vi "nanocal -- nuclear schottky fit V7.vi"() -> ()   [LabVIEW 2021] (continued)
0.000000000000   ,  \"Imoff\" -> 0.000000000000   ,  \"στ1\" -> 0.000000000000   ,  \"στS\" -> 0.000000000000   ,  \"στN\" -> 0.000000000000    |>   , \n\"IDS0531_220605_RAW_cal__ref_\" ->   <|    \"ζ\" -> 0.047292360430   ,  \"τ1\" -> 0.215650832524   ,  \"τS\" -> 0.021748628873   ,  \"τN\" -> 0.002014257649   ,  \"τC\" -> 0.001656178311   ,  \"κ0\" -> 0.000000003034   ,  \"mm1\" -> 0.000069918264   ,  \"mm2\" -> 0.024098100915   ,  \"mm3\" -> 0.218025681173   ,  \"T\" -> 0.520000000000   ,  \"B\" -> 4.000000000000   ,  \"θ\" -> 45.000000000000   ,  \"Reoff\" -> -2955102.040816321970   ,  \"Imoff\" -> 0.000000000000   ,  \"στ1\" -> 0.046963197390   ,  \"στS\" -> 0.000145543572   ,  \"στN\" -> 0.000181922698    |>   , \n\"IDS0531_220605_RAW_cal__sam_\" ->   <|    \"ζ\" -> 0.000000000000   ,  \"τ1\" -> 0.000000000000   ,  \"τS\" -> 0.000000000000   ,  \"τN\" -> 0.000000000000   ,  \"τC\" -> 0.000000000000   ,  \"κ0\" -> 0.000000000000   ,  \"mm1\" -> 0.000000000000   ,  \"mm2\" -> 0.000000000000   ,  \"mm3\" -> 0.000000000000   ,  \"T\" -> 0.520000000000   ,  \"B\" -> 4.000000000000   ,  \"θ\" -> 45.000000000000   ,  \"Reoff\" -> 0.000000000000   ,  \"Imoff\" -> 0.000000000000   ,  \"στ1\" -> 0.000000000000   ,  \"στS\" -> 0.000000000000   ,  \"στN\" -> 0.000000000000    |>   , \n\"IDS0532_220605_RAW_cal__ref_\" ->   <|    \"ζ\" -> 0.039581980273   ,  \"τ1\" -> 0.217269361754   ,  \"τS\" -> 0.023071327438   ,  \"τN\" -> 0.001182618434   ,  \"τC\" -> 0.001652851775   ,  \"κ0\" -> 0.000000003717   ,  \"mm1\" -> 0.000059010683   ,  \"mm2\" -> 0.025415535832   ,  \"mm3\" -> 0.218661632092   ,  \"T\" -> 0.620000000000   ,  \"B\" -> 4.000000000000   ,  \"θ\" -> 45.000000000000   ,  \"Reoff\" -> -2746938.775510199370   ,  \"Imoff\" -> 0.000000000000   ,  \"στ1\" -> 0.015098698436   ,  \"στS\" -> 0.000189797573   ,  \"στN\" -> 0.000008998512    |>   , \n\"IDS0532_220605_RAW_cal__sam_\" ->   <|    \"ζ\" -> 0.000000000000   ,  \"τ1\" -> 0.000000000000   ,  \"τS\" -> 0.000000000000   ,  \"τN\" -> 0.000000000000   ,  \"τC\" -> 0.000000000000   ,  \"κ0\" -> 0.000000000000   ,  \"mm1\" -> 0.000000000000   ,  \"mm2\" -> 0.000000000000   ,  \"mm3\" -> 0.000000000000   ,  \"T\" -> 0.620000000000   ,  \"B\" -> 4.000000000000   ,  \"θ\" -> 45.000000000000   ,  \"Reoff\" -> 0.000000000000   ,  \"Imoff\" -> 0.000000000000   ,  \"στ1\" -> 0.000000000000   ,  \"στS\" -> 0.000000000000   ,  \"στN\" -> 0.000000000000    |>   , \n\"IDS0533_220605_RAW_cal__ref_\" ->   <|    \"ζ\" -> 0.026006399704   ,  \"τ1\" -> 0.219491604326   ,  \"τS\" -> 0.026508960211   ,  \"τN\" -> 0.000691251356   ,  \"τC\" -> 0.002192117759   ,  \"κ0\" -> 0.000000005099   ,  \"mm1\" -> 0.000051510023   ,  \"mm2\" -> 0.029230026409   ,  \"mm3\" -> 0.220309776794   ,  \"T\" -> 0.820000000000   ,  \"B\" -> 4.000000000000   ,  \"θ\" -> 45.000000000000   ,  \"Reoff\" -> -873469.387755103408   ,  \"Imoff\" -> 0.000000000000   ,  \"στ1\" -> 0.040897544111   ,  \"στS\" -> 0.000189265066   ,  \"στN\" -> 0.000022111002    |>   , \n\"IDS0533_220605_RAW_cal__sam_\" ->   <|    \"ζ\" -> 0.000000000000   ,  \"τ1\" -> 0.000000000000   ,  \"τS\" -> 0.000000000000   ,  \"τN\" -> 0.000000000000   ,  \"τC\" -> 0.000000000000   ,  \"κ0\" -> 0.000000000000   ,  \"mm1\" -> 0.000000000000   ,  \"mm2\" -> 0.000000000000   ,  \"mm3\" -> 0.000000000000   ,  \"T\" -> 0.820000000000   ,  \"B\" -> 4.000000000000   ,  \"θ\" -> 45.000000000000   ,  \"Reoff\" -> 0.000000000000   ,  \"Imoff\" -> 0.000000000000   ,  \"στ1\" -> 0.000000000000   ,  \"στS\" -> 0.000000000000   ,  \"στN\" -> 0.000000000000    |>   , \n\"IDS0534_220605_RAW_cal__ref_\" ->   <|    \"ζ\" -> 0.022451049934   ,  \"τ1\" -> 0.221358754558   ,  \"τS\" -> 0.033966694492   ,  \"τN\" -> 0.000363309481   ,  \"τC\" -> 0.002245679298   ,  \"κ0\" -> 0.000000007138   ,  \"mm1\" -> 0.000046374039   ,  \"mm2\" -> 0.036854393963   ,  \"mm3\" -> 0.221804414461   ,  \"T\" -> 1.120000000000   ,  \"B\" -> 4.000000000000   ,  \"θ\" -> 45.000000000000   ,  \"Reoff\" -> -885714.285714285447   ,  \"Imoff\" -> 0.000000000000   ,  \"στ1\" -> 0.023144908767   ,  \"στS\" -> 0.000217300505   ,  \"στN\" -> 0.000007634517    |>   , \n\"IDS0534_220605_RAW_cal__sam_\" ->   <|    \"ζ\" -> 0.000000000000   ,  \"τ1\" -> 0.000000000000   ,  \"τS\" -> 0.000000000000   ,  \"τN\" -> 0.000000000000   ,  \"τC\" -> 0.000000000000   ,  \"κ0\" -> 0.000000000000   ,  \"mm1\" -> 0.000000000000   ,  \"mm2\" -> 0.000000000000   ,  \"mm3\" -> 0.000000000000   ,  \"T\" -> 1.120000000000   ,  \"B\" -> 4.000000000000   ,  \"θ\" -> 45.000000000000   ,  \"Reoff\" -> 0.000000000000   ,  \"Imoff\" -> 0.000000000000   ,  \"στ1\" -> 0.000000000000   ,  \"στS\" -> 0.000000000000   ,  \"στN\" -> 0.000000000000    |>   , \n\"IDS0535_220605_RAW_cal__ref_\" ->   <|    \"ζ\" -> 0.019576865757   ,  \"τ1\" -> 0.218088277374   ,  \"τS\" -> 0.022473990539   ,  \"τN\" -> 0.000172254737   ,  \"τC\" -> 0.002442141955   ,  \"κ0\" -> 0.000000011417   ,  \"mm1\" -> 0.000042446249   ,  \"mm2\" -> 0.025290622371   ,  \"mm3\" -> 0.218286938488   ,  \"T\" -> 1.700000000000   ,  \"B\" -> 4.000000000000   ,  \"θ\" -> 45.000000000000   ,  \"Reoff\" -> -322448.979591836221   ,  \"Imoff\" -> 0.000000000000   ,  \"στ1\" -> 0.063627358635   ,  \"στS\" -> 0.000720787697   ,  \"στN\" -> 0.000014224220    |>   , \n\"IDS0535_220605_RAW_cal__sam_\" ->   <|    \"ζ\" -> 0.000000000000   ,  \"τ1\" -> 0.000000000000   ,  \"τS\" -> 0.000000000000   ,  \"τN\" -> 0.000000000000   ,  \"τC\" -> 0.000000000000   ,  \"κ0\" -> 0.000000000000   ,  \"mm1\" -> 0.000000000000   ,  \"mm2\" -> 0.000000000000   ,  \"mm3\" -> 0.000000000000   ,  \"T\" -> 1.700000000000   ,  \"B\" -> 4.000000000000   ,  \"θ\" -> 45.000000000000   ,  \"Reoff\" -> 0.000000000000   ,  \"Imoff\" -> 0.000000000000   ,  \"στ1\" -> 0.000000000000   ,  \"στS\" -> 0.000000000000   ,  \"στN\" -> 0.000000000000    |>   , \n\"IDS0536_220605_RAW_cal__ref_\" ->   <|    \"ζ\" -> 0.017203827920   ,  \"τ1\" -> 0.213925239716   ,  \"τS\" -> 0.013557235716   ,  \"τN\" -> 0.000118116880   ,  \"τC\" -> 0.002620828700   ,  \"κ0\" -> 0.000000012687   ,  \"mm1\" -> 0.000037331962   ,  \"mm2\" -> 0.016364021106   ,  \"mm3\" -> 0.214055336357   ,  \"T\" -> 1.900000000000   ,  \"B\" -> 4.000000000000   ,  \"θ\" -> 45.000000000000   ,  \"Reoff\" -> -322448.979591836221   ,  \"Imoff\" -> 0.000000000000   ,  \"στ1\" -> 0.007920167579   ,  \"στS\" -> 0.000110474044   ,  \"στN\" -> 0.000002075732    |>   , \n\"IDS0536_220605_RAW_cal__sam_\" ->   <|    \"ζ\" -> 0.000000000000   ,  \"τ1\" -> 0.000000000000   ,  \"τS\" -> 0.000000000000   ,  \"τN\" -> 0.000000000000   ,  \"τC\" -> 0.000000000000   ,  \"κ0\" -> 0.000000000000   ,  \"mm1\" -> 0.000000000000   ,  \"mm2\" -> 0.000000000000   ,  \"mm3\" -> 0.000000000000   ,  \"T\" -> 1.900000000000   ,  \"B\" -> 4.000000000000   ,  \"θ\" -> 45.000000000000   ,  \"Reoff\" -> 0.000000000000   ,  \"Imoff\" -> 0.000000000000   ,  \"στ1\" -> 0.000000000000   ,  \"στS\" -> 0.000000000000   ,  \"στN\" -> 0.000000000000    |>   , \n\"IDS0537_220605_RAW_cal__ref_\" ->   <|    \"ζ\" -> 0.016837588937   ,  \"τ1\" -> 0.214083726987   ,  \"τS\" -> 0.009462256875   ,  \"τN\" -> 0.000044961797   ,  \"τC\" -> 0.002520072033   ,  \"κ0\" -> 0.000000022492   ,  \"mm1\" -> 0.000033158698   ,  \"mm2\" -> 0.012105753537   ,  \"mm3\" -> 0.214132184097   ,  \"T\" -> 3.100000000000   ,  \"B\" -> 4.000000000000   ,  \"θ\" -> 45.000000000000   ,  \"Reoff\" -> -200000.000000000000   ,  \"Imoff\" -> 0.000000000000   ,  \"στ1\" -> 0.041355363203   ,  \"στS\" -> 0.000204828997   ,  \"στN\" -> 0.000003281967    |>   , \n\"IDS0537_220605_RAW_cal__sam_\" ->   <|    \"ζ\" -> 0.000000000000   ,  \"τ1\" -> 0.000000000000   ,  \"τS\" -> 0.000000000000   ,  \"τN\" -> 0.000000000000   ,  \"τC\" -> 0.000000000000   ,  \"κ0\" -> 0.000000000000   ,  \"mm1\" -> 0.000000000000   ,  \"mm2\" -> 0.000000000000   ,  \"mm3\" -> 0.000000000000   ,  \"T\" -> 3.100000000000   ,  \"B\" -> 4.000000000000   ,  \"θ\" -> 45.000000000000   ,  \"Reoff\" -> 0.000000000000   ,  \"Imoff\" -> 0.000000000000   ,  \"στ1\" -> 0.000000000000   ,  \"στS\" -> 0.000000000000   ,  \"στN\" -> 0.000000000000    |>   , \n\"IDS0538_220605_RAW_cal__ref_\" ->   <|    \"ζ\" -> 0.019986975905   ,  \"τ1\" -> 0.213955272188   ,  \"τS\" -> 0.005937059985   ,  \"τN\" -> 0.000017131866   ,  \"τC\" -> 0.001979607590   ,  \"κ0\" -> 0.000000055230   ,  \"mm1\" -> 0.000029341516   ,  \"mm2\" -> 0.008005311507   ,  \"mm3\" -> 0.213973424895   ,  \"T\" -> 5.700000000000   ,  \"B\" -> 4.000000000000   ,  \"θ\" -> 45.000000000000   ,  \"Reoff\" -> -77551.020408162847   ,  \"Imoff\" -> 0.000000000000   ,  \"στ1\" -> 0.013237190857   ,  \"στS\" -> 0.000032983186   ,  \"στN\" -> 0.000000229969    |>   , \n\"IDS0538_220605_RAW_cal__sam_\" ->   <|    \"ζ\" -> 0.000000000000   ,  \"τ1\" -> 0.000000000000   ,  \"τS\" -> 0.000000000000   ,  \"τN\" -> 0.000000000000   ,  \"τC\" -> 0.000000000000   ,  \"κ0\" -> 0.000000000000   ,  \"mm1\" -> 0.000000000000   ,  \"mm2\" -> 0.000000000000   ,  \"mm3\" -> 0.000000000000   ,  \"T\" -> 5.700000000000   ,  \"B\" -> 4.000000000000   ,  \"θ\" -> 45.000000000000   ,  \"Reoff\" -> 0.000000000000   ,  \"Imoff\" -> 0.000000000000   ,  \"στ1\" -> 0.000000000000   ,  \"στS\" -> 0.000000000000   ,  \"στN\" -> 0.000000000000    |>   , \n\"IDS0540_220605_RAW_cal__ref_\" ->   <|    \"ζ\" -> 0.251392330354   ,  \"τ1\" -> 0.346377607558   ,  \"τS\" -> 0.016513842206   ,  \"τN\" -> 0.014262469720   ,  \"τC\" -> 0.000857308117   ,  \"κ0\" -> 0.000000000886   ,  \"mm1\" -> 0.000166652692   ,  \"mm2\" -> 0.020248144591   ,  \"mm3\" -> 0.365333359092   ,  \"T\" -> 0.200000000000   ,  \"B\" -> 2.000000000000   ,  \"θ\" -> 45.000000000000   ,  \"Reoff\" -> -46204081.632653057600   ,  \"Imoff\" -> 0.000000000000   ,  \"στ1\" -> 0.424749382693   ,  \"στS\" -> 0.000332071104   ,  \"στN\" -> 0.013507044944    |>   , \n\"IDS0540_220605_RAW_cal__sam_\" ->   <|    \"ζ\" -> 0.000000000000   ,  \"τ1\" -> 0.000000000000   ,  \"τS\" -> 0.000000000000   ,  \"τN\" -> 0.000000000000   ,  \"τC\" -> 0.000000000000   ,  \"κ0\" -> 0.000000000000   ,  \"mm1\" -> 0.000000000000   ,  \"mm2\" -> 0.000000000000   ,  \"mm3\" -> 0.000000000000   ,  \"T\" -> 0.200000000000   ,  \"B\" -> 2.000000000000   ,  \"θ\" -> 45.000000000000   ,  \"Reoff\" -> 0.000000000000   ,  \"Imoff\" -> 0.000000000000   ,  \"στ1\" -> 0.000000000000   ,  \"στS\" -> 0.000000000000   ,  \"στN\" -> 0.000000000000    |>   , \n\"IDS0541_220605_RAW_cal__ref_\" ->   <|    \"ζ\" -> 0.165113897347   ,  \"τ1\" -> 0.387980452993   ,  \"τS\" -> 0.014374929410   ,  \"τN\" -> 0.009383556190   ,  \"τC\" -> 0.000942269686   ,  \"κ0\" -> 0.000000001199   ,  \"mm1\" -> 0.000127336399   ,  \"mm2\" -> 0.017060680127   ,  \"mm3\" -> 0.399416047906   ,  \"T\" -> 0.250000000000   ,  \"B\" -> 2.000000000000   ,  \"θ\" -> 45.000000000000   ,  \"Reoff\" -> -23306122.448979616200   ,  \"Imoff\" -> 0.000000000000   ,  \"στ1\" -> 0.067668625614   ,  \"στS\" -> 0.000112915267   ,  \"στN\" -> 0.002227405906    |>   , \n\"IDS0541_220605_RAW_cal__sam_\" ->   <|    \"ζ\" -> 0.000000000000   ,  \"τ1\" -> 0.000000000000   ,  \"τS\" -> 0.000000000000   ,  \"τN\" -> 0.000000000000   ,  \"τC\" -> 0.000000000000   ,  \"κ0\" -> 0.000000000000   ,  \"mm1\" -> 0.000000000000   ,  \"mm2\" -> 0.000000000000   ,  \"mm3\" -> 0.000000000000   ,  \"T\" -> 0.250000000000   ,  \"B\" -> 2.000000000000   ,  \"θ\" -> 45.000000000000   ,  \"Reoff\" -> 0.000000000000   ,  \"Imoff\" -> 0.000000000000   ,  \"στ1\" -> 0.000000000000   ,  \"στS\" -> 0.000000000000   ,  \"στN\" -> 0.000000000000    |>   , \n\"IDS0542_220606_RAW_cal__ref_\" ->   <|    \"ζ\" -> 0.345710784026   ,  \"τ1\" -> 0.327857477320   ,  \"τS\" -> 0.019203362427   ,  \"τN\" -> 0.016889536551   ,  \"τC\" -> 0.000830598267   ,  \"κ0\" -> 0.000000000695   ,  \"mm1\" -> 0.000208359489   ,  \"mm2\" -> 0.024619495516   ,  \"mm3\" -> 0.352430823963   ,  \"T\" -> 0.170000000000   ,  \"B\" -> 2.000000000000   ,  \"θ\" -> 45.000000000000   ,  \"Reoff\" -> -73265306.122448980800   ,  \"Imoff\" -> 0.000000000000   ,  \"στ1\" -> 0.369953882310   ,  \"στS\" -> 0.000610690630   ,  \"στN\" -> 0.016945730597    |>   , \n\"IDS0542_220606_RAW_cal__sam_\" ->   <|    \"ζ\" -> 0.000000000000   ,  \"τ1\" -> 0.000000000000   ,  \"τS\" -> 0.000000000000   ,  \"τN\" -> 0.000000000000   ,  \"τC\" -> 0.000000000000   ,  \"κ0\" -> 0.000000000000   ,  \"mm1\" -> 0.000000000000   ,  \"mm2\" -> 0.000000000000   ,  \"mm3\" -> 0.000000000000   ,  \"T\" -> 0.170000000000   ,  \"B\" -> 2.000000000000   ,  \"θ\" -> 45.000000000000   ,  \"Reoff\" -> 0.000000000000   ,  \"Imoff\" -> 0.000000000000   ,  \"στ1\" -> 0.000000000000   ,  \"στS\" -> 0.000000000000   ,  \"στN\" -> 0.000000000000    |>   , \n\"IDS0543_220606_RAW_cal__ref_\" ->   <|    \"ζ\" -> 0.443467990428   ,  \"τ1\" -> 0.317886288494   ,  \"τS\" -> 0.021647161508   ,  \"τN\" -> 0.018036346988   ,  \"τC\" -> 0.000838651939   ,  \"κ0\" -> 0.000000000590   ,  \"mm1\" -> 0.000252909908   ,  \"mm2\" -> 0.029199801325   ,  \"mm3\" -> 0.346554103461   ,  \"T\" -> 0.150000000000   ,  \"B\" -> 2.000000000000   ,  \"θ\" -> 45.000000000000   ,  \"Reoff\" -> -94081632.653061270700   ,  \"Imoff\" -> 0.000000000000   ,  \"στ1\" -> 0.633667064980   ,  \"στS\" -> 0.001327852543   ,  \"στN\" -> 0.033112841100    |>   , \n\"IDS0543_220606_RAW_cal__sam_\" ->   <|    \"ζ\" -> 0.000000000000   ,  \"τ1\" -> 0.000000000000   ,  \"τS\" -> 0.000000000000   ,  \"τN\" -> 0.000000000000   ,  \"τC\" -> 0.000000000000   ,  \"κ0\" -> 0.000000000000   ,  \"mm1\" -> 0.000000000000   ,  \"mm2\" -> 0.000000000000   ,  \"mm3\" -> 0.000000000000   ,  \"T\" -> 0.150000000000   ,  \"B\" -> 2.000000000000   ,  \"θ\" -> 45.000000000000   ,  \"Reoff\" -> 0.000000000000   ,  \"Imoff\" -> 0.000000000000   ,  \"στ1\" -> 0.000000000000   ,  \"στS\" -> 0.000000000000   ,  \"στN\" -> 0.000000000000    |>   , \n\"IDS0544_220606_RAW_cal__ref_\" ->   <|    \"ζ\" -> 0.664244638441   ,  \"τ1\" -> 0.246856024037   ,  \"τS\" -> 0.027685516986   ,  \"τN\" -> 0.022864655649   ,  \"τC\" -> 0.000854076829   ,  \"κ0\" -> 0.000000000436   ,  \"mm1\" -> 0.000337098347   ,  \"mm2\" -> 0.039372294078   ,  \"mm3\" -> 0.292128562221   ,  \"T\" -> 0.120000000000   ,  \"B\" -> 2.000000000000   ,  \"θ\" -> 45.000000000000   ,  \"Reoff\" -> -183040816.326530635000   ,  \"Imoff\" -> 0.000000000000   ,  \"στ1\" -> 0.607479321028   ,  \"στS\" -> 0.003421096587   ,  \"στN\" -> 0.047598917320    |>   , \n\"IDS0544_220606_RAW_cal__sam_\" ->   <|    \"ζ\" -> 0.000000000000   ,  \"τ1\" -> 0.000000000000   ,  \"τS\" -> 0.000000000000   ,  \"τN\" -> 0.000000000000   ,  \"τC\" -> 0.000000000000   ,  \"κ0\" -> 0.000000000000   ,  \"mm1\" -> 0.000000000000   ,  \"mm2\" -> 0.000000000000   ,  \"mm3\" -> 0.000000000000   ,  \"T\" -> 0.120000000000   ,  \"B\" -> 2.000000000000   ,  \"θ\" -> 45.000000000000   ,  \"Reoff\" -> 0.000000000000   ,  \"Imoff\" -> 0.000000000000   ,  \"στ1\" -> 0.000000000000   ,  \"στS\" -> 0.000000000000   ,  \"στN\" -> 0.000000000000    |>   , \n\"IDS0545_220606_RAW_cal__ref_\" ->   <|    \"ζ\" -> 0.114584837195   ,  \"τ1\" -> 0.375837377440   ,  \"τS\" -> 0.013356599543   ,  \"τN\" -> 0.007350942831   ,  \"τC\" -> 0.001154352119   ,  \"κ0\" -> 0.000000001547   ,  \"mm1\" -> 0.000110898808   ,  \"mm2\" -> 0.015576445529   ,  \"mm3\" -> 0.384384697967   ,  \"T\" -> 0.300000000000   ,  \"B\" -> 2.000000000000   ,  \"θ\" -> 45.000000000000   ,  \"Reoff\" -> -9836734.693877555430   ,  \"Imoff\" -> 0.000000000000   ,  \"στ1\" -> 0.036231793577   ,  \"στS\" -> 0.000070867254   ,  \"στN\" -> 0.000621210167    |>   , \n\"IDS0545_220606_RAW_cal__sam_\" ->   <|    \"ζ\" -> 0.000000000000   ,  \"τ1\" -> 0.000000000000   ,  \"τS\" -> 0.000000000000   ,  \"τN\" -> 0.000000000000   ,  \"τC\" -> 0.000000000000   ,  \"κ0\" -> 0.000000000000   ,  \"mm1\" -> 0.000000000000   ,  \"mm2\" -> 0.000000000000   ,  \"mm3\" -> 0.000000000000   ,  \"T\" -> 0.300000000000   ,  \"B\" -> 2.000000000000   ,  \"θ\" -> 45.000000000000   ,  \"Reoff\" -> 0.000000000000   ,  \"Imoff\" -> 0.000000000000   ,  \"στ1\" -> 0.000000000000   ,  \"στS\" -> 0.000000000000   ,  \"στN\" -> 0.000000000000    |>   , \n\"IDS0546_220606_RAW_cal__ref_\" ->   <|    \"ζ\" -> 0.086559942010   ,  \"τ1\" -> 0.376689726376   ,  \"τS\" -> 0.013025220586   ,  \"τN\" -> 0.006974345540   ,  \"τC\" -> 0.001217354577   ,  \"κ0\" -> 0.000000001917   ,  \"mm1\" -> 0.000089822592   ,  \"mm2\" -> 0.014966812259   ,  \"mm3\" -> 0.384581173512   ,  \"T\" -> 0.360000000000   ,  \"B\" -> 2.000000000000   ,  \"θ\" -> 45.000000000000   ,  \"Reoff\" -> -8612244.897959187630   ,  \"Imoff\" -> 0.000000000000   ,  \"στ1\" -> 0.438938204284   ,  \"στS\" -> 0.000131885488   ,  \"στN\" -> 0.003309064048    |>   , \n\"IDS0546_220606_RAW_cal__sam_\" ->   <|    \"ζ\" -> 0.000000000000   ,  \"τ1\" -> 0.000000000000   ,  \"τS\" -> 0.000000000000   ,  \"τN\" -> 0.000000000000   ,  \"τC\" -> 0.000000000000   ,  \"κ0\" -> 0.000000000000   ,  \"mm1\" -> 0.000000000000   ,  \"mm2\" -> 0.000000000000   ,  \"mm3\" -> 0.000000000000   ,  \"T\" -> 0.360000000000   ,  \"B\" -> 2.000000000000   ,  \"θ\" -> 45.000000000000   ,  \"Reoff\" -> 0.000000000000   ,  \"Imoff\" -> 0.000000000000   ,  \"στ1\" -> 0.000000000000   ,  \"στS\" -> 0.000000000000   ,  \"στN\" -> 0.000000000000    |>   , \n\"IDS0547_220606_RAW_cal__ref_\" ->   <|    \"ζ\" -> 0.069999106625   ,  \"τ1\" -> 0.375220053416   ,  \"τS\" -> 0.013216291389   ,  \"τN\" -> 0.005647516312   ,  \"τC\" -> 0.001254063929   ,  \"κ0\" -> 0.000000002317   ,  \"mm1\" -> 0.000075729851   ,  \"mm2\" -> 0.015067056915   ,  \"mm3\" -> 0.381515587966   ,  \"T\" -> 0.420000000000   ,  \"B\" -> 2.000000000000   ,  \"θ\" -> 45.000000000000   ,  \"Reoff\" -> -7142857.142857141800   ,  \"Imoff\" -> 0.000000000000   ,  \"στ1\" -> 0.247259195832   ,  \"στS\" -> 0.000163525957   ,  \"στN\" -> 0.005342009137    |>   , \n\"IDS0547_220606_RAW_cal__sam_\" ->   <|    \"ζ\" -> 0.000000000000   ,  \"τ1\" -> 0.000000000000   ,  \"τS\" -> 0.000000000000   ,  \"τN\" -> 0.000000000000   ,  \"τC\" -> 0.000000000000   ,  \"κ0\" -> 0.000000000000   ,  \"mm1\" -> 0.000000000000   ,  \"mm2\" -> 0.000000000000   ,  \"mm3\" -> 0.000000000000   ,  \"T\" -> 0.420000000000   ,  \"B\" -> 2.000000000000   ,  \"θ\" -> 45.000000000000   ,  \"Reoff\" -> 0.000000000000   ,  \"Imoff\" -> 0.000000000000   ,  \"στ1\" -> 0.000000000000   ,  \"στS\" -> 0.000000000000   ,  \"στN\" -> 0.000000000000    |>   , \n\"IDS0548_220606_RAW_cal__ref_\" ->   <|    \"ζ\" -> 0.050401769736   ,  \"τ1\" -> 0.373876419184   ,  \"τS\" -> 0.013977187329   ,  \"τN\" -> 0.005482355270   ,  \"τC\" -> 0.001501801590   ,  \"κ0\" -> 0.000000002989   ,  \"mm1\" -> 0.000065640074   ,  \"mm2\" -> 0.015862773261   ,  \"mm3\" -> 0.379890145424   ,  \"T\" -> 0.520000000000   ,  \"B\" -> 2.000000000000   ,  \"θ\" -> 45.000000000000   ,  \"Reoff\" -> -3714285.714285716420   ,  \"Imoff\" -> 0.000000000000   ,  \"στ1\" -> 0.110713266907   ,  \"στS\" -> 0.000122907745   ,  \"στN\" -> 0.001966965268    |>   , \n\"IDS0548_220606_RAW_cal__sam_\" ->   <|    \"ζ\" -> 0.000000000000   ,  \"τ1\" -> 0.000000000000   ,  \"τS\" -> 0.000000000000   ,  \"τN\" -> 0.000000000000   ,  \"τC\" -> 0.000000000000   ,  \"κ0\" -> 0.000000000000   ,  \"mm1\" -> 0.000000000000   ,  \"mm2\" -> 0.000000000000   ,  \"mm3\" -> 0.000000000000   ,  \"T\" -> 0.520000000000   ,  \"B\" -> 2.000000000000   ,  \"θ\" -> 45.000000000000   ,  \"Reoff\" -> 0.000000000000   ,  \"Imoff\" -> 0.000000000000   ,  \"στ1\" -> 0.000000000000   ,  \"στS\" -> 0.000000000000   ,  \"στN\" -> 0.000000000000    |>   , \n\"IDS0549_220606_RAW_cal__ref_\" ->   <|    \"ζ\" -> 0.041979401075   ,  \"τ1\" -> 0.368478793966   ,  \"τS\" -> 0.015446799439   ,  \"τN\" -> 0.003402337716   ,  \"τC\" -> 0.001575093876   ,  \"κ0\" -> 0.000000003686   ,  \"mm1\" -> 0.000057991267   ,  \"mm2\" -> 0.017436315900   ,  \"mm3\" -> 0.372199993318   ,  \"T\" -> 0.620000000000   ,  \"B\" -> 2.000000000000   ,  \"θ\" -> 45.000000000000   ,  \"Reoff\" -> -2979591.836734697220   ,  \"Imoff\" -> 0.000000000000   ,  \"στ1\" -> 0.135403699680   ,  \"στS\" -> 0.000163058440   ,  \"στN\" -> 0.001967445367    |>   , \n\"IDS0550_220606_RAW_cal__ref_\" ->   <|    \"ζ\" -> 0.030650031864   ,  \"τ1\" -> 0.371061825507   ,  \"τS\" -> 0.019434774268   ,  \"τN\" -> 0.003191687976   ,  \"τC\" -> 0.001854354331   ,  \"κ0\" -> 0.000000005040   ,  \"mm1\" -> 0.000050590010   ,  \"mm2\" -> 0.021630629169   ,  \"mm3\" -> 0.374554924692   ,  \"T\" -> 0.820000000000   ,  \"B\" -> 2.000000000000   ,  \"θ\" -> 45.000000000000   ,  \"Reoff\" -> -1632653.061224489940   ,  \"Imoff\" -> 0.000000000000   ,  \"στ1\" -> 0.107047861270   ,  \"στS\" -> 0.000201030582   ,  \"στN\" -> 0.000503414357    |>   , \n\"IDS0550_220606_RAW_cal__sam_\" ->   <|    \"ζ\" -> 0.000000000000   ,  \"τ1\" -> 0.000000000000   ,  \"τS\" -> 0.000000000000   ,  \"τN\" -> 0.000000000000   ,  \"τC\" -> 0.000000000000   ,  \"κ0\" -> 0.000000000000   ,  \"mm1\" -> 0.000000000000   ,  \"mm2\" -> 0.000000000000   ,  \"mm3\" -> 0.000000000000   ,  \"T\" -> 0.820000000000   ,  \"B\" -> 2.000000000000   ,  \"θ\" -> 45.000000000000   ,  \"Reoff\" -> 0.000000000000   ,  \"Imoff\" -> 0.000000000000   ,  \"στ1\" -> 0.000000000000   ,  \"στS\" -> 0.000000000000   ,  \"στN\" -> 0.000000000000    |>   , \n\"IDS0551_220606_RAW_cal__ref_\" ->   <|    \"ζ\" -> 0.023490949621   ,  \"τ1\" -> 0.378878569703   ,  \"τS\" -> 0.026968462806   ,  \"τN\" -> 0.001819085143   ,  \"τC\" -> 0.002360831644   ,  \"κ0\" -> 0.000000007142   ,  \"mm1\" -> 0.000049999340   ,  \"mm2\" -> 0.029754158704   ,  \"mm3\" -> 0.380899038091   ,  \"T\" -> 1.120000000000   ,  \"B\" -> 2.000000000000   ,  \"θ\" -> 45.000000000000   ,  \"Reoff\" -> -959183.673469387924   ,  \"Imoff\" -> 0.000000000000   ,  \"στ1\" -> 0.190596529331   ,  \"στS\" -> 0.000292683710   ,  \"στN\" -> 0.000959345989    |>   , \n\"IDS0551_220606_RAW_cal__sam_\" ->   <|    \"ζ\" -> 0.000000000000   ,  \"τ1\" -> 0.000000000000   ,  \"τS\" -> 0.000000000000   ,  \"τN\" -> 0.000000000000   ,  \"τC\" -> 0.000000000000   ,  \"κ0\" -> 0.000000000000   ,  \"mm1\" -> 0.000000000000   ,  \"mm2\" -> 0.000000000000   ,  \"mm3\" -> 0.000000000000   ,  \"T\" -> 1.120000000000   ,  \"B\" -> 2.000000000000   ,  \"θ\" -> 45.000000000000   ,  \"Reoff\" -> 0.000000000000   ,  \"Imoff\" -> 0.000000000000   ,  \"στ1\" -> 0.000000000000   ,  \"στS\" -> 0.000000000000   ,  \"στN\" -> 0.000000000000    |>   , \n\"IDS0552_220606_RAW_cal__ref_\" ->   <|    \"ζ\" -> 0.016903896176   ,  \"τ1\" -> 0.389208085767   ,  \"τS\" -> 0.042839293805   ,  \"τN\" -> 0.001054381509   ,  \"τC\" -> 0.002700942117   ,  \"κ0\" -> 0.000000012752   ,  \"mm1\" -> 0.000042315056   ,  \"mm2\" -> 0.046078096141   ,  \"mm3\" -> 0.390424266131   ,  \"T\" -> 1.900000000000   ,  \"B\" -> 2.000000000000   ,  \"θ\" -> 45.000000000000   ,  \"Reoff\" -> -285714.285714285448   ,  \"Imoff\" -> 0.000000000000   ,  \"στ1\" -> 0.071680793743   ,  \"στS\" -> 0.000751471945   ,  \"στN\" -> 0.000020808748    |>   , \n\"IDS0552_220606_RAW_cal__sam_\" ->   <|    \"ζ\" -> 0.000000000000   ,  \"τ1\" -> 0.000000000000   ,  \"τS\" -> 0.000000000000   ,  \"τN\" -> 0.000000000000   ,  \"τC\" -> 0.000000000000   ,  \"κ0\" -> 0.000000000000   ,  \"mm1\" -> 0.000000000000   ,  \"mm2\" -> 0.000000000000   ,  \"mm3\" -> 0.000000000000   ,  \"T\" -> 1.900000000000   ,  \"B\" -> 2.000000000000   ,  \"θ\" -> 45.000000000000   ,  \"Reoff\" -> 0.000000000000   ,  \"Imoff\" -> 0.000000000000   ,  \"στ1\" -> 0.000000000000   ,  \"στS\" -> 0.000000000000   ,  \"στN\" -> 0.000000000000    |>   , \n\"IDS0553_220606_RAW_cal__ref_\" ->   <|    \"ζ\" -> 0.019034298387   ,  \"τ1\" -> 0.340685747660   ,  \"τS\" -> 0.012600728873   ,  \"τN\" -> 0.000836062096   ,  \"τC\" -> 0.002405907399   ,  \"κ0\" -> 0.000000015790   ,  \"mm1\" -> 0.000037942280   ,  \"mm2\" -> 0.015168856864   ,  \"mm3\" -> 0.341577406773   ,  \"T\" -> 2.300000000000   ,  \"B\" -> 2.000000000000   ,  \"θ\" -> 45.000000000000   ,  \"Reoff\" -> -346938.775510204024   ,  \"Imoff\" -> 0.000000000000   ,  \"στ1\" -> 0.043118413730   ,  \"στS\" -> 0.000142443187   ,  \"στN\" -> 0.000023036701    |>   , \n\"IDS0553_220606_RAW_cal__sam_\" ->   <|    \"ζ\" -> 0.000000000000   ,  \"τ1\" -> 0.000000000000   ,  \"τS\" -> 0.000000000000   ,  \"τN\" -> 0.000000000000   ,  \"τC\" -> 0.000000000000   ,  \"κ0\" -> 0.000000000000   ,  \"mm1\" -> 0.000000000000   ,  \"mm2\" -> 0.000000000000   ,  \"mm3\" -> 0.000000000000   ,  \"T\" -> 2.300000000000   ,  \"B\" -> 2.000000000000   ,  \"θ\" -> 45.000000000000   ,  \"Reoff\" -> 0.000000000000   ,  \"Imoff\" -> 0.000000000000   ,  \"στ1\" -> 0.000000000000   ,  \"στS\" -> 0.000000000000   ,  \"στN\" -> 0.000000000000    |>   , \n\"IDS0554_220606_RAW_cal__ref_\" ->   <|    \"ζ\" -> 0.019434711880   ,  \"τ1\" -> 0.338729084958   ,  \"τS\" -> 0.009688878082   ,  \"τN\" -> 0.000475618163   ,  \"τC\" -> 0.002360170204   ,  \"κ0\" -> 0.000000022449   ,  \"mm1\" -> 0.000036425186   ,  \"mm2\" -> 0.012182847072   ,  \"mm3\" -> 0.339232023205   ,  \"T\" -> 3.100000000000   ,  \"B\" -> 2.000000000000   ,  \"θ\" -> 45.000000000000   ,  \"Reoff\" -> -224489.795918367803   ,  \"Imoff\" -> 0.000000000000   ,  \"στ1\" -> 0.018790484107   ,  \"στS\" -> 0.000064367566   ,  \"στN\" -> 0.000007244630    |>   , \n\"IDS0554_220606_RAW_cal__sam_\" ->   <|    \"ζ\" -> 0.000000000000   ,  \"τ1\" -> 0.000000000000   ,  \"τS\" -> 0.000000000000   ,  \"τN\" -> 0.000000000000   ,  \"τC\" -> 0.000000000000   ,  \"κ0\" -> 0.000000000000   ,  \"mm1\" -> 0.000000000000   ,  \"mm2\" -> 0.000000000000   ,  \"mm3\" -> 0.000000000000   ,  \"T\" -> 3.100000000000   ,  \"B\" -> 2.000000000000   ,  \"θ\" -> 45.000000000000   ,  \"Reoff\" -> 0.000000000000   ,  \"Imoff\" -> 0.000000000000   ,  \"στ1\" -> 0.000000000000   ,  \"στS\" -> 0.000000000000   ,  \"στN\" -> 0.000000000000    |>   , \n\"IDS0555_220606_RAW_cal__ref_\" ->   <|    \"ζ\" -> 0.021952381066   ,  \"τ1\" -> 0.337915266866   ,  \"τS\" -> 0.005864517957   ,  \"τN\" -> 0.000285674383   ,  \"τC\" -> 0.001869482382   ,  \"κ0\" -> 0.000000055591   ,  \"mm1\" -> 0.000030729933   ,  \"mm2\" -> 0.007825098033   ,  \"mm3\" -> 0.338214124988   ,  \"T\" -> 5.700000000000   ,  \"B\" -> 2.000000000000   ,  \"θ\" -> 45.000000000000   ,  \"Reoff\" -> -102040.816326530650   ,  \"Imoff\" -> 0.000000000000   ,  \"στ1\" -> 0.018966360272   ,  \"στS\" -> 0.000034456720   ,  \"στN\" -> 0.000003385178    |>   , \n\"IDS0555_220606_RAW_cal__sam_\" ->   <|    \"ζ\" -> 0.000000000000   ,  \"τ1\" -> 0.000000000000   ,  \"τS\" -> 0.000000000000   ,  \"τN\" -> 0.000000000000   ,  \"τC\" -> 0.000000000000   ,  \"κ0\" -> 0.000000000000   ,  \"mm1\" -> 0.000000000000   ,  \"mm2\" -> 0.000000000000   ,  \"mm3\" -> 0.000000000000   ,  \"T\" -> 5.700000000000   ,  \"B\" -> 2.000000000000   ,  \"θ\" -> 45.000000000000   ,  \"Reoff\" -> 0.000000000000   ,  \"Imoff\" -> 0.000000000000   ,  \"στ1\" -> 0.000000000000   ,  \"στS\" -> 0.000000000000   ,  \"στN\" -> 0.000000000000    |>   , \n\"IDS0556_220606_RAW_cal__ref_\" ->   <|    \"ζ\" -> 0.018774663118   ,  \"τ1\" -> 0.223771999883   ,  \"τS\" -> 0.042172507139   ,  \"τN\" -> 0.000220913712   ,  \"τC\" -> 0.002321380026   ,  \"κ0\" -> 0.000000009770   ,  \"mm1\" -> 0.000040623453   ,  \"mm2\" -> 0.045188092517   ,  \"mm3\" -> 0.224054006985   ,  \"T\" -> 1.500000000000   ,  \"B\" -> 4.000000000000   ,  \"θ\" -> 45.000000000000   ,  \"Reoff\" -> -530612.244897959753   ,  \"Imoff\" -> 0.000000000000   ,  \"στ1\" -> 0.017095464532   ,  \"στS\" -> 0.000347466214   ,  \"στN\" -> 0.000004822339    |>   , \n\"IDS0556_220606_RAW_cal__sam_\" ->   <|    \"ζ\" -> 0.000000000000   ,  \"τ1\" -> 0.000000000000   ,  \"τS\" -> 0.000000000000   ,  \"τN\" -> 0.000000000000   ,  \"τC\" -> 0.000000000000   ,  \"κ0\" -> 0.000000000000   ,  \"mm1\" -> 0.000000000000   ,  \"mm2\" -> 0.000000000000   ,  \"mm3\" -> 0.000000000000   ,  \"T\" -> 1.500000000000   ,  \"B\" -> 4.000000000000   ,  \"θ\" -> 45.000000000000   ,  \"Reoff\" -> 0.000000000000   ,  \"Imoff\" -> 0.000000000000   ,  \"στ1\" -> 0.000000000000   ,  \"στS\" -> 0.000000000000   ,  \"στN\" -> 0.000000000000    |>   , \n\"IDS0559_220607_RAW_cal__ref_\" ->   <|    \"ζ\" -> 0.355714515528   ,  \"τ1\" -> 0.301914651842   ,  \"τS\" -> 0.015251938720   ,  \"τN\" -> 0.009436044938   ,  \"τC\" -> 0.000785444302   ,  \"κ0\" -> 0.000000000710   ,  \"mm1\" -> 0.000200413404   ,  \"mm2\" -> 0.020338541635   ,  \"mm3\" -> 0.315630998909   ,  \"T\" -> 0.170000000000   ,  \"B\" -> 2.000000000000   ,  \"θ\" -> 0.000000000000   ,  \"Reoff\" -> -74000000.000000000000   ,  \"Imoff\" -> 0.000000000000   ,  \"στ1\" -> 0.232297531792   ,  \"στS\" -> 0.000374376394   ,  \"στN\" -> 0.007678585568    |>   , \n\"IDS0559_220607_RAW_cal__sam_\" ->   <|    \"ζ\" -> 0.000000000000   ,  \"τ1\" -> 0.000000000000   ,  \"τS\" -> 0.000000000000   ,  \"τN\" -> 0.000000000000   ,  \"τC\" -> 0.000000000000   ,  \"κ0\" -> 0.000000000000   ,  \"mm1\" -> 0.000000000000   ,  \"mm2\" -> 0.000000000000   ,  \"mm3\" -> 0.000000000000   ,  \"T\" -> 0.170000000000   ,  \"B\" -> 2.000000000000   ,  \"θ\" -> 0.000000000000   ,  \"Reoff\" -> 0.000000000000   ,  \"Imoff\" -> 0.000000000000   ,  \"στ1\" -> 0.000000000000   ,  \"στS\" -> 0.000000000000   ,  \"στN\" -> 0.000000000000    |>   , \n\"IDS0560_220607_RAW_cal__ref_\" ->   <|    \"ζ\" -> 0.449635679893   ,  \"τ1\" -> 0.299060701269   ,  \"τS\" -> 0.016808041703   ,  \"τN\" -> 0.012305660826   ,  \"τC\" -> 0.000825775215   ,  \"κ0\" -> 0.000000000592   ,  \"mm1\" -> 0.000250217726   ,  \"mm2\" -> 0.023425417691   ,  \"mm3\" -> 0.318415103028   ,  \"T\" -> 0.150000000000   ,  \"B\" -> 2.000000000000   ,  \"θ\" -> 0.000000000000   ,  \"Reoff\" -> -98857142.857142850800   ,  \"Imoff\" -> 0.000000000000   ,  \"στ1\" -> 1.839545255469   ,  \"στS\" -> 0.000824368006   ,  \"στN\" -> 0.069201981467    |>   , \n\"IDS0560_220607_RAW_cal__sam_\" ->   <|    \"ζ\" -> 0.000000000000   ,  \"τ1\" -> 0.000000000000   ,  \"τS\" -> 0.000000000000   ,  \"τN\" -> 0.000000000000   ,  \"τC\" -> 0.000000000000   ,  \"κ0\" -> 0.000000000000   ,  \"mm1\" -> 0.000000000000   ,  \"mm2\" -> 0.000000000000   ,  \"mm3\" -> 0.000000000000   ,  \"T\" -> 0.150000000000   ,  \"B\" -> 2.000000000000   ,  \"θ\" -> 0.000000000000   ,  \"Reoff\" -> 0.000000000000   ,  \"Imoff\" -> 0.000000000000   ,  \"στ1\" -> 0.000000000000   ,  \"στS\" -> 0.000000000000   ,  \"στN\" -> 0.000000000000    |>   , \n\"IDS0561_220607_RAW_cal__ref_\" ->   <|    \"ζ\" -> 0.668963686378   ,  \"τ1\" -> 0.239112055774   ,  \"τS\" -> 0.021396471169   ,  \"τN\" -> 0.016347037663   ,  \"τC\" -> 0.000866848111   ,  \"κ0\" -> 0.000000000434   ,  \"mm1\" -> 0.000342420854   ,  \"mm2\" -> 0.032017103471   ,  \"mm3\" -> 0.270611925197   ,  \"T\" -> 0.120000000000   ,  \"B\" -> 2.000000000000   ,  \"θ\" -> 0.000000000000   ,  \"Reoff\" -> -192285714.285714298000   ,  \"Imoff\" -> 0.000000000000   ,  \"στ1\" -> 1.100347031208   ,  \"στS\" -> 0.002027710728   ,  \"στN\" -> 0.065388411976    |>   , \n\"IDS0561_220607_RAW_cal__sam_\" ->   <|    \"ζ\" -> 0.000000000000   ,  \"τ1\" -> 0.000000000000   ,  \"τS\" -> 0.000000000000   ,  \"τN\" -> 0.000000000000   ,  \"τC\" -> 0.000000000000   ,  \"κ0\" -> 0.000000000000   ,  \"mm1\" -> 0.000000000000   ,  \"mm2\" -> 0.000000000000   ,  \"mm3\" -> 0.000000000000   ,  \"T\" -> 0.120000000000   ,  \"B\" -> 2.000000000000   ,  \"θ\" -> 0.000000000000   ,  \"Reoff\" -> 0.000000000000   ,  \"Imoff\" -> 0.000000000000   ,  \"στ1\" -> 0.000000000000   ,  \"στS\" -> 0.000000000000   ,  \"στN\" -> 0.000000000000    |>   , \n\"IDS0562_220607_RAW_cal__ref_\" ->   <|    \"ζ\" -> 0.258991387788   ,  \"τ1\" -> 0.317151511252   ,  \"τS\" -> 0.013390047800   ,  \"τN\" -> 0.006328285333   ,  \"τC\" -> 0.000848770466   ,  \"κ0\" -> 0.000000000905   ,  \"mm1\" -> 0.000167822844   ,  \"mm2\" -> 0.017085435691   ,  \"mm3\" -> 0.325572234779   ,  \"T\" -> 0.200000000000   ,  \"B\" -> 2.000000000000   ,  \"θ\" -> 0.000000000000   ,  \"Reoff\" -> -44857142.857142865700   ,  \"Imoff\" -> 0.000000000000   ,  \"στ1\" -> 0.531664595642   ,  \"στS\" -> 0.000229891647   ,  \"στN\" -> 0.006046488522    |>   , \n\"IDS0562_220607_RAW_cal__sam_\" ->   <|    \"ζ\" -> 0.000000000000   ,  \"τ1\" -> 0.000000000000   ,  \"τS\" -> 0.000000000000   ,  \"τN\" -> 0.000000000000   ,  \"τC\" -> 0.000000000000   ,  \"κ0\" -> 0.000000000000   ,  \"mm1\" -> 0.000000000000   ,  \"mm2\" -> 0.000000000000   ,  \"mm3\" -> 0.000000000000   ,  \"T\" -> 0.200000000000   ,  \"B\" -> 2.000000000000   ,  \"θ\" -> 0.000000000000   ,  \"Reoff\" -> 0.000000000000   ,  \"Imoff\" -> 0.000000000000   ,  \"στ1\" -> 0.000000000000   ,  \"στS\" -> 0.000000000000   ,  \"στN\" -> 0.000000000000    |>   , \n\"IDS0563_220607_RAW_cal__ref_\" ->   <|    \"ζ\" -> 0.172150656876   ,  \"τ1\" -> 0.349830224606   ,  \"τS\" -> 0.011998498670   ,  \"τN\" -> 0.004489980914   ,  \"τC\" -> 0.000896743670   ,  \"κ0\" -> 0.000000001200   ,  \"mm1\" -> 0.000124849196   ,  \"mm2\" -> 0.014606727837   ,  \"mm3\" -> 0.355322373419   ,  \"T\" -> 0.250000000000   ,  \"B\" -> 2.000000000000   ,  \"θ\" -> 0.000000000000   ,  \"Reoff\" -> -26000000.000000000000   ,  \"Imoff\" -> 0.000000000000   ,  \"στ1\" -> 0.049625629402   ,  \"στS\" -> 0.000087536047   ,  \"στN\" -> 0.000631838919    |>   , \n\"IDS0563_220607_RAW_cal__sam_\" ->   <|    \"ζ\" -> 0.000000000000   ,  \"τ1\" -> 0.000000000000   ,  \"τS\" -> 0.000000000000   ,  \"τN\" -> 0.000000000000   ,  \"τC\" -> 0.000000000000   ,  \"κ0\" -> 0.000000000000   ,  \"mm1\" -> 0.000000000000   ,  \"mm2\" -> 0.000000000000   ,  \"mm3\" -> 0.000000000000   ,  \"T\" -> 0.250000000000   ,  \"B\" -> 2.000000000000   ,  \"θ\" -> 0.000000000000   ,  \"Reoff\" -> 0.000000000000   ,  \"Imoff\" -> 0.000000000000   ,  \"στ1\" -> 0.000000000000   ,  \"στS\" -> 0.000000000000   ,  \"στN\" -> 0.000000000000    |>   , \n\"IDS0564_220607_RAW_cal__ref_\" ->   <|    \"ζ\" -> 0.118516574313   ,  \"τ1\" -> 0.350390004709   ,  \"τS\" -> 0.011220444254   ,  \"τN\" -> 0.003404891640   ,  \"τC\" -> 0.001143718862   ,  \"κ0\" -> 0.000000001568   ,  \"mm1\" -> 0.000111980338   ,  \"mm2\" -> 0.013430301860   ,  \"mm3\" -> 0.354350121975   ,  \"T\" -> 0.300000000000   ,  \"B\" -> 2.000000000000   ,  \"θ\" -> 0.000000000000   ,  \"Reoff\" -> -11428571.428571432800   ,  \"Imoff\" -> 0.000000000000   ,  \"στ1\" -> 0.301334297831   ,  \"στS\" -> 0.000157213626   ,  \"στN\" -> 0.004248705404    |>   , \n\"IDS0564_220607_RAW_cal__sam_\" ->   <|    \"ζ\" -> 0.000000000000   ,  \"τ1\" -> 0.000000000000   ,  \"τS\" -> 0.000000000000   ,  \"τN\" -> 0.000000000000   ,  \"τC\" -> 0.000000000000   ,  \"κ0\" -> 0.000000000000   ,  \"mm1\" -> 0.000000000000   ,  \"mm2\" -> 0.000000000000   ,  \"mm3\" -> 0.000000000000   ,  \"T\" -> 0.300000000000   ,  \"B\" -> 2.000000000000   ,  \"θ\" -> 0.000000000000   ,  \"Reoff\" -> 0.000000000000   ,  \"Imoff\" -> 0.000000000000   ,  \"στ1\" -> 0.000000000000   ,  \"στS\" -> 0.000000000000   ,  \"στN\" -> 0.000000000000    |>   , \n\"IDS0565_220607_RAW_cal__ref_\" ->   <|    \"ζ\" -> 0.087986482080   ,  \"τ1\" -> 0.256186322762   ,  \"τS\" -> 0.011079357499   ,  \"τN\" -> 0.003568927376   ,  \"τC\" -> 0.001270661793   ,  \"κ0\" -> 0.000000001939   ,  \"mm1\" -> 0.000093617177   ,  \"mm2\" -> 0.013023417519   ,  \"mm3\" -> 0.260277085788   ,  \"T\" -> 0.360000000000   ,  \"B\" -> 2.000000000000   ,  \"θ\" -> 0.000000000000   ,  \"Reoff\" -> -8000000.000000000000   ,  \"Imoff\" -> 0.000000000000   ,  \"στ1\" -> 0.066076122842   ,  \"στS\" -> 0.000113449498   ,  \"στN\" -> 0.000256105794    |>   , \n\"IDS0565_220607_RAW_cal__sam_\" ->   <|    \"ζ\" -> 0.000000000000   ,  \"τ1\" -> 0.000000000000   ,  \"τS\" -> 0.000000000000   ,  \"τN\" -> 0.000000000000   ,  \"τC\" -> 0.000000000000   ,  \"κ0\" -> 0.000000000000   ,  \"mm1\" -> 0.000000000000   ,  \"mm2\" -> 0.000000000000   ,  \"mm3\" -> 0.000000000000   ,  \"T\" -> 0.360000000000   ,  \"B\" -> 2.000000000000   ,  \"θ\" -> 0.000000000000   ,  \"Reoff\" -> 0.000000000000   ,  \"Imoff\" -> 0.000000000000   ,  \"στ1\" -> 0.000000000000   ,  \"στS\" -> 0.000000000000   ,  \"στN\" -> 0.000000000000    |>   , \n\"IDS0566_220607_RAW_cal__ref_\" ->   <|    \"ζ\" -> 0.070156403527   ,  \"τ1\" -> 0.262147223577   ,  \"τS\" -> 0.011262923295   ,  \"τN\" -> 0.002364637934   ,  \"τC\" -> 0.001329677258   ,  \"κ0\" -> 0.000000002344   ,  \"mm1\" -> 0.000078974457   ,  \"mm2\" -> 0.013170019334   ,  \"mm3\" -> 0.264811528958   ,  \"T\" -> 0.420000000000   ,  \"B\" -> 2.000000000000   ,  \"θ\" -> 0.000000000000   ,  \"Reoff\" -> -6285714.285714268690   ,  \"Imoff\" -> 0.000000000000   ,  \"στ1\" -> 0.014203019449   ,  \"στS\" -> 0.000120077801   ,  \"στN\" -> 0.000048266431    |>   , \n\"IDS0566_220607_RAW_cal__sam_\" ->   <|    \"ζ\" -> 0.000000000000   ,  \"τ1\" -> 0.000000000000   ,  \"τS\" -> 0.000000000000   ,  \"τN\" -> 0.000000000000   ,  \"τC\" -> 0.000000000000   ,  \"κ0\" -> 0.000000000000   ,  \"mm1\" -> 0.000000000000   ,  \"mm2\" -> 0.000000000000   ,  \"mm3\" -> 0.000000000000   ,  \"T\" -> 0.420000000000   ,  \"B\" -> 2.000000000000   ,  \"θ\" -> 0.000000000000   ,  \"Reoff\" -> 0.000000000000   ,  \"Imoff\" -> 0.000000000000   ,  \"στ1\" -> 0.000000000000   ,  \"στS\" -> 0.000000000000   ,  \"στN\" -> 0.000000000000    |>   , \n\"IDS0567_220607_RAW_cal__ref_\" ->   <|    \"ζ\" -> 0.052694231594   ,  \"τ1\" -> 0.206237698748   ,  \"τS\" -> 0.012180702952   ,  \"τN\" -> 0.001670150721   ,  \"τC\" -> 0.001358485752   ,  \"κ0\" -> 0.000000003021   ,  \"mm1\" -> 0.000061755571   ,  \"mm2\" -> 0.013991387047   ,  \"mm3\" -> 0.208123755646   ,  \"T\" -> 0.520000000000   ,  \"B\" -> 2.000000000000   ,  \"θ\" -> 0.000000000000   ,  \"Reoff\" -> -4571428.571428567170   ,  \"Imoff\" -> 0.000000000000   ,  \"στ1\" -> 0.013542176029   ,  \"στS\" -> 0.000128345810   ,  \"στN\" -> 0.000027133680    |>   , \n\"IDS0567_220607_RAW_cal__sam_\" ->   <|    \"ζ\" -> 0.000000000000   ,  \"τ1\" -> 0.000000000000   ,  \"τS\" -> 0.000000000000   ,  \"τN\" -> 0.000000000000   ,  \"τC\" -> 0.000000000000   ,  \"κ0\" -> 0.000000000000   ,  \"mm1\" -> 0.000000000000   ,  \"mm2\" -> 0.000000000000   ,  \"mm3\" -> 0.000000000000   ,  \"T\" -> 0.520000000000   ,  \"B\" -> 2.000000000000   ,  \"θ\" -> 0.000000000000   ,  \"Reoff\" -> 0.000000000000   ,  \"Imoff\" -> 0.000000000000   ,  \"στ1\" -> 0.000000000000   ,  \"στS\" -> 0.000000000000   ,  \"στN\" -> 0.000000000000    |>   , \n\"IDS0568_220607_RAW_cal__ref_\" ->   <|    \"ζ\" -> 0.042136652692   ,  \"τ1\" -> 0.203636345776   ,  \"τS\" -> 0.013404195797   ,  \"τN\" -> 0.001074940238   ,  \"τC\" -> 0.001728340244   ,  \"κ0\" -> 0.000000003726   ,  \"mm1\" -> 0.000062435783   ,  \"mm2\" -> 0.015542386487   ,  \"mm3\" -> 0.204849102111   ,  \"T\" -> 0.620000000000   ,  \"B\" -> 2.000000000000   ,  \"θ\" -> 0.000000000000   ,  \"Reoff\" -> -2612244.897959183900   ,  \"Imoff\" -> 0.000000000000   ,  \"στ1\" -> 0.011688220611   ,  \"στS\" -> 0.000121966623   ,  \"στN\" -> 0.000019089189    |>   , \n\"IDS0568_220607_RAW_cal__sam_\" ->   <|    \"ζ\" -> 0.000000000000   ,  \"τ1\" -> 0.000000000000   ,  \"τS\" -> 0.000000000000   ,  \"τN\" -> 0.000000000000   ,  \"τC\" -> 0.000000000000   ,  \"κ0\" -> 0.000000000000   ,  \"mm1\" -> 0.000000000000   ,  \"mm2\" -> 0.000000000000   ,  \"mm3\" -> 0.000000000000   ,  \"T\" -> 0.620000000000   ,  \"B\" -> 2.000000000000   ,  \"θ\" -> 0.000000000000   ,  \"Reoff\" -> 0.000000000000   ,  \"Imoff\" -> 0.000000000000   ,  \"στ1\" -> 0.000000000000   ,  \"στS\" -> 0.000000000000   ,  \"στN\" -> 0.000000000000    |>   , \n\"IDS0569_220607_RAW_cal__ref_\" ->   <|    \"ζ\" -> 0.030235387858   ,  \"τ1\" -> 0.200849812033   ,  \"τS\" -> 0.016889405709   ,  \"τN\" -> 0.000765333865   ,  \"τC\" -> 0.002360193521   ,  \"κ0\" -> 0.000000005110   ,  \"mm1\" -> 0.000061183035   ,  \"mm2\" -> 0.019613778642   ,  \"mm3\"
